vi "sampling1.vi"() -> ()   [LabVIEW 2017]
panel:
  out "Frequency 2":dbl
  out "Amplitude 2":dbl
  in  "Duration (s)":dbl=1.0
  out "Waveform Graph 2":dynamicdata(graph)
  out "Waveform Graph":dynamicdata(graph)
  in  "Frequency":dbl=1000.0
  in  "Amplitude":dbl=2.0
  # "This Waveform graph show \nthe waveform of the signal"
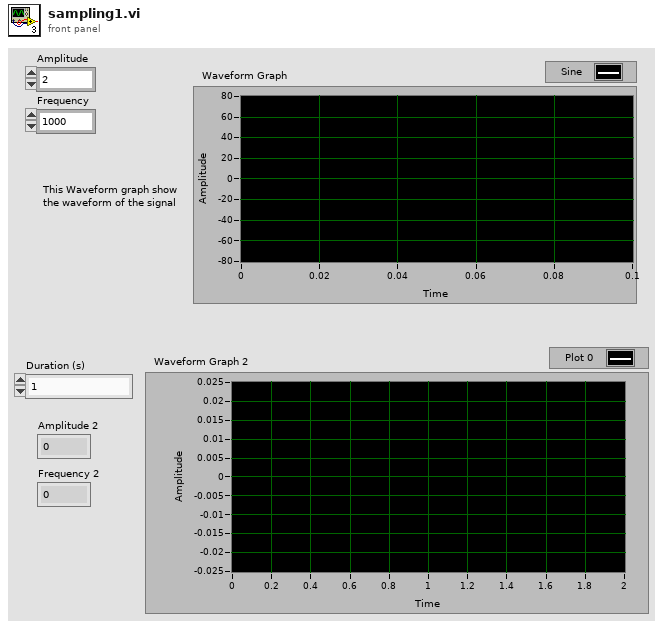
[diagram p1: front panel]
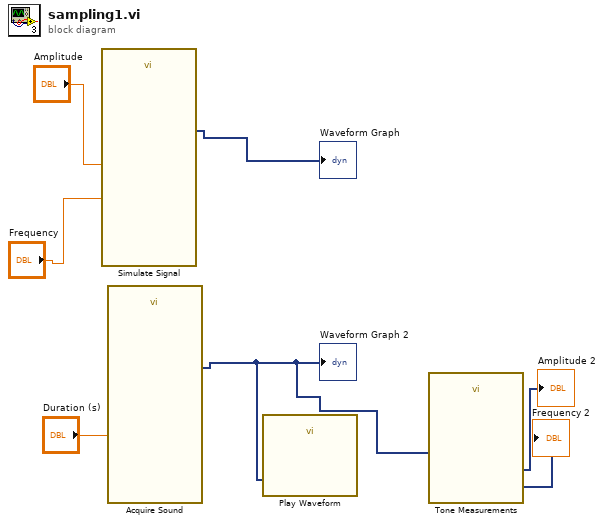
[diagram p0: block diagram]
diagram:
  n1 = call "Simulate Signal"("Frequency"="Frequency", "Amplitude"="Amplitude") -> ("Sine"=→"Waveform Graph":dynamicdata)  [unwired: 12 in, 1 out]
  n2 = call "Acquire Sound"("Duration (s)"="Duration (s)") -> ("Data"=w3:dynamicdata)  [unwired: 17 in, 1 out]
  "Waveform Graph 2" <- w3
  n3 = call "Play Waveform"("Data"=w3) -> ()  [unwired: 18 in, 1 out]
  n4 = call "Tone Measurements"("Signals"=w3) -> ("Frequency"=→"Frequency 2":dynamicdata, "Amplitude"=→"Amplitude 2":dynamicdata)  [unwired: 8 in, 1 out]
